vi "fftwf_memcpy_to_cplx.vi"(8 "error in (no error)":errorcluster, 10 "cplx count":i32, 11 "*data_in":u64) -> (0 "error out":errorcluster, 2 "cplx sgl array out":csg[](array[numeric]), 3 "*data_in (copy)":u64)   [LabVIEW 2020, in "FFTWDLL.lvlib"]
doc: "Copy FFTW cplx single data to LV CSGL array."
uses:
  FFTWDLL.lvlib
  ntdll.dll
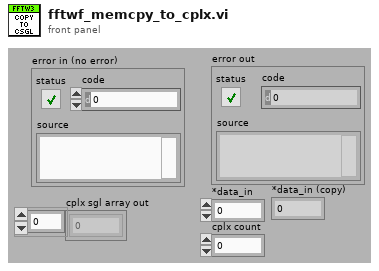
[diagram p1: front panel]
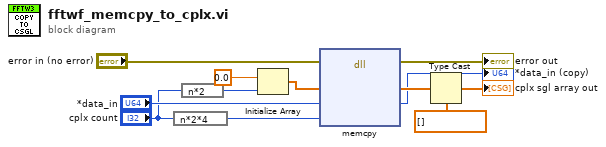
[diagram p0: block diagram]
diagram:
  n1 = expression code="n*2*4"("cplx count") -> (w10:i32)
  n2 = expression code="n*2"("cplx count") -> (w5:i32)
  n3 = Initialize Array(sgl 0.0, w5) -> (w8:sgl[])
  n4 = dll-call lib="ntdll.dll" fn="memcpy"(error in="error in (no error)", "dest"=w8, "src"="*data_in", "n"=w10) -> (error out=→"error out":errorcluster, "dest"=w4:sgl[], "src"=→"*data_in (copy)":i64)  [unwired: 4 in, 1 out]
  n5 = Type Cast(type=csg[] [], x=w4) -> (*(type *) &x=→"cplx sgl array out":csg[])
